vi "Add Pattern Script Header.vi"(8 "error in (no error)":errorcluster, 9 "Pattern Script Frame in":string, 10 "Pattern Name":string, 11 "SPI Root Pattern Creator in":refnum<class "SPI Root Pattern Creator.lvclass">) -> (0 "error out":errorcluster, 2 "Pattern Script All out":string, 3 "SPI Root Pattern Creator out":refnum<class "SPI Root Pattern Creator.lvclass">)   [LabVIEW 2018, in "SPI Root Pattern Creator.lvlib" / "SPI Root Pattern Creator.lvclass"]
uses:
  SPI Root Pattern Creator.lvclass
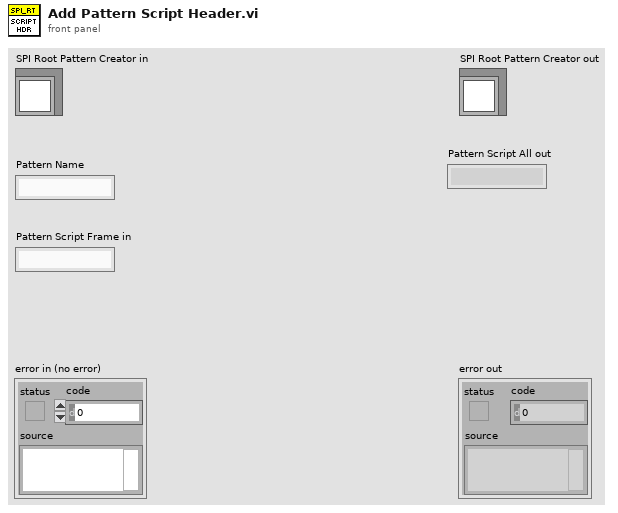
[diagram p1: front panel]
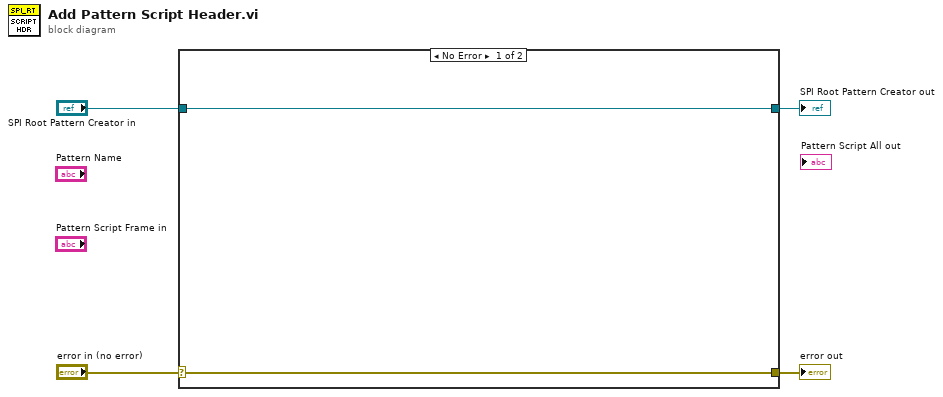
[diagram p0: block diagram]
diagram:
  n1 = case shown="No Error" "error in (no error)" {
    selector: "error in (no error)" -> [w5 w8]
    tunnel: [w5 w8] -> w3
    tunnel: [w6 w7] -> w1
    tunnel: "SPI Root Pattern Creator in" -> [w6 w7]
    frame No Error {
    }
    frame Error {
    }
  }
  "error out" <- w3
  "SPI Root Pattern Creator out" <- w1
